vi "All Tests.vi"() -> (0 "error out":errorcluster)   [LabVIEW 2020, in "Unit Tests.lvlib"]
uses:
  Unit Tests.lvlib
  <vilib>/addons/_JKI Toolkits/Caraya/classes/Test Suite/Test Suite.lvclass
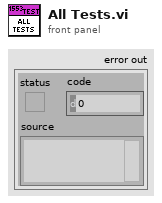
[diagram p1: front panel]
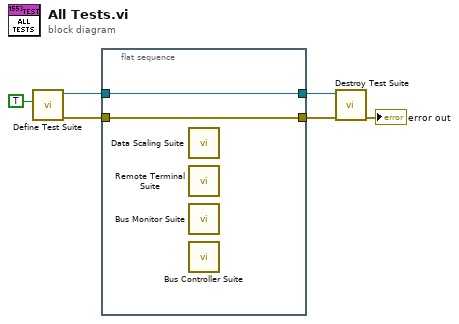
[diagram p0: block diagram]
diagram:
  n1 = call <vilib>:"Define Test Suite.vi"("Interactive"=TRUE) -> ("error out"=w3:errorcluster, "Test Suite"=w5:refnum<class "Test Suite.lvclass">)  [unwired: 8 in, 1 out]
  n2 = flat-sequence {
    tunnel: [w8] -> w6
    tunnel: w5 -> [w8]
    tunnel: [w7] -> w4
    tunnel: w3 -> [w7]
    frame #0 {
      n3 = call "Data Scaling Suite.vi"() -> ()  [unwired: 12 in]
      n4 = call "Remote Terminal Suite.vi"() -> ()  [unwired: 12 in]
      n5 = call "Bus Monitor Suite.vi"() -> ()  [unwired: 12 in]
      n6 = call "Bus Controller Suite.vi"() -> ()  [unwired: 12 in]
    }
  }
  n7 = call-dynamic "Destroy Test Suite.vi"("error in (no error)"=w4, "Test Suite in"=w6) -> ("error out"=→"error out":errorcluster)  [unwired: 8 in, 1 out]
